vi "Info.vi"(7 "Message":string, 8 "error in (no error)":errorcluster, 11 "Logger in":refnum<class "Logger.lvclass">) -> (0 "error out":errorcluster, 3 "Logger out":refnum<class "Logger.lvclass">)   [LabVIEW 2022 SP3, in "Logger.lvlib" / "Logger.lvclass"]
uses:
  Logger.lvclass
  PythonWrapper/Source/PythonSession/PythonSession.lvclass/PythonSession.ctl
  PythonWrapper/Source/PythonWrapper/PythonWrapper.lvclass/PythonWrapper.ctl
  LoggingWrapper/LoggingWrapper.lvclass/LoggingWrapper.ctl
  Logger.lvclass/Logger.ctl
  PythonWrapper/Source/PythonSession/Read PythonSession.vi
  PythonWrapper/Source/PythonWrapper/Read ModulePath.vi
  Read Name.vi
  PythonWrapper/Source/PythonSession/SessionBank.vi
  _Level.ctl
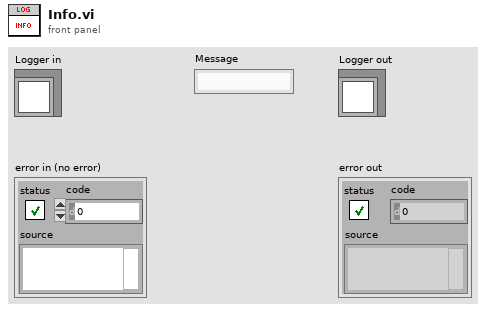
[diagram p1: front panel]
types:
  T1 = typedef "Logger.lvlib/Logger.lvclass/_Level.ctl" = enum16{"NOTSET", "DEBUG", "INFO", "WARNING", "ERROR", "CRITICAL"}
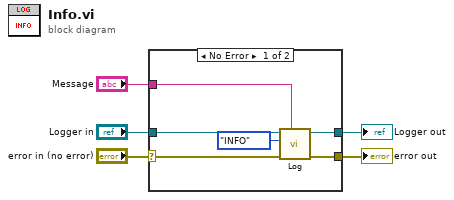
[diagram p0: block diagram]
diagram:
  n1 = case shown="No Error" "error in (no error)" {
    selector: "error in (no error)" -> [w11 w13]
    tunnel: [w10 w13] -> w1
    tunnel: [w8 w12] -> w3
    tunnel: "Logger in" -> [w9 w12]
    tunnel: "Message" -> [w7 _]
    frame No Error {
      n2 = call-dynamic "Log.vi"("Message"=w7, "error in (no error)"=w11, "Level"=_Level."INFO", "Logger in"=w9) -> ("error out"=w10:errorcluster, "Logger out"=w8:refnum<class "Logger.lvclass">)  [unwired: 6 in]
    }
    frame Error {
    }
  }
  "error out" <- w1
  "Logger out" <- w3
